vi "Get Lvm Data.vi"(8 "Error In":errorcluster, 11 "Path In":path) -> (0 "Error Out":errorcluster, 2 "Traces":T1(array[cluster]), 3 "Path Out":path)   [LabVIEW 2014, in "Aquisicao de Dados.lvlib"]
uses:
  Aquisicao de Dados.lvlib
  <vilib>/regexp/Match Regular Expression.xnode
panel:
  out "Waveform Graph":waveform(dbl)[](graph)
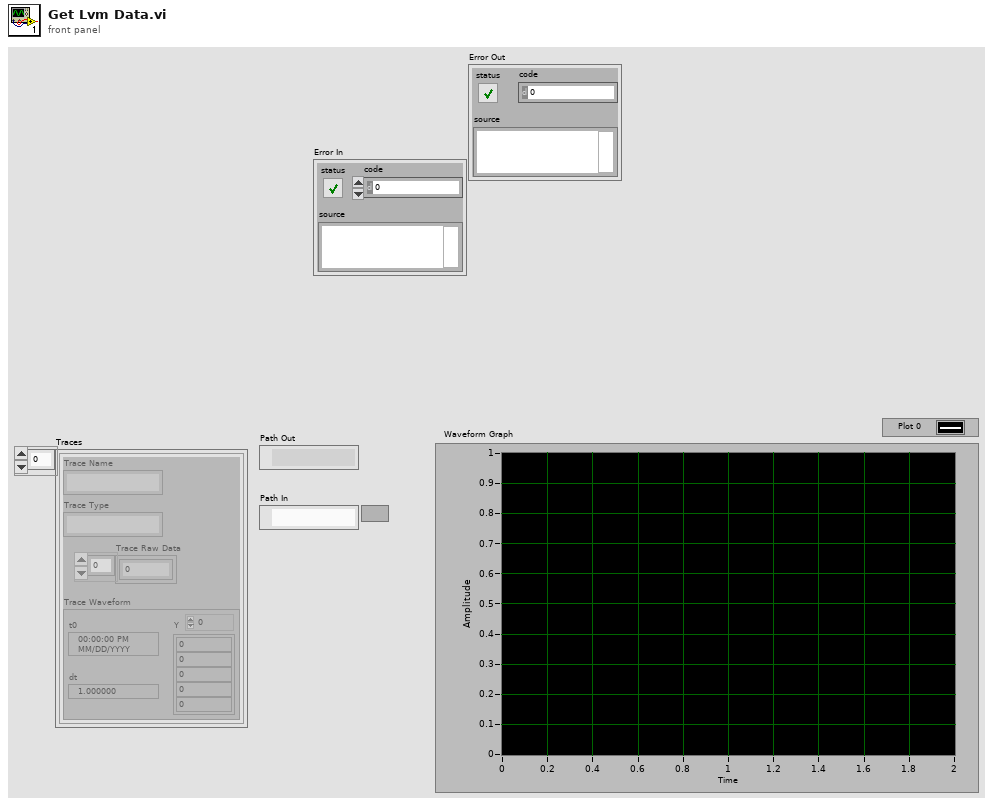
[diagram p1: front panel]
types:
  T1 = cluster{"Trace Name":string, "Trace Type":string, "Trace Raw Data":dbl[], "Trace Waveform":waveform(dbl)}[]
  T2 = cluster{"Trace Name":string, "Trace Type":string, "Trace Raw Data":dbl[], "Trace Waveform":waveform(dbl)}
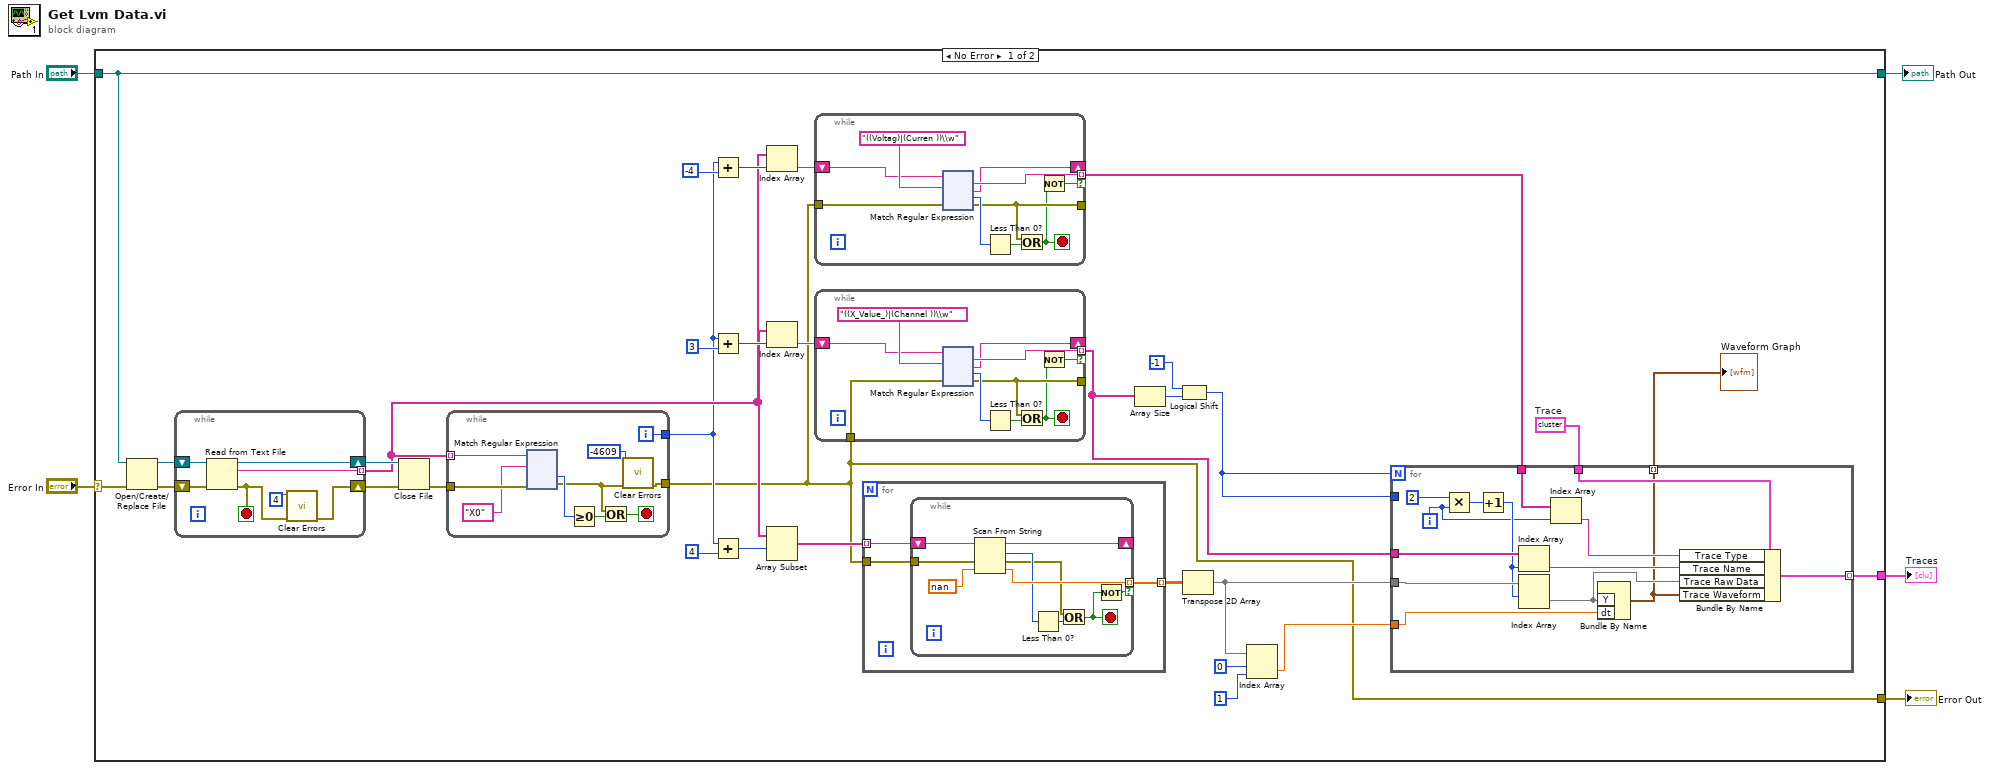
[diagram p0: block diagram]
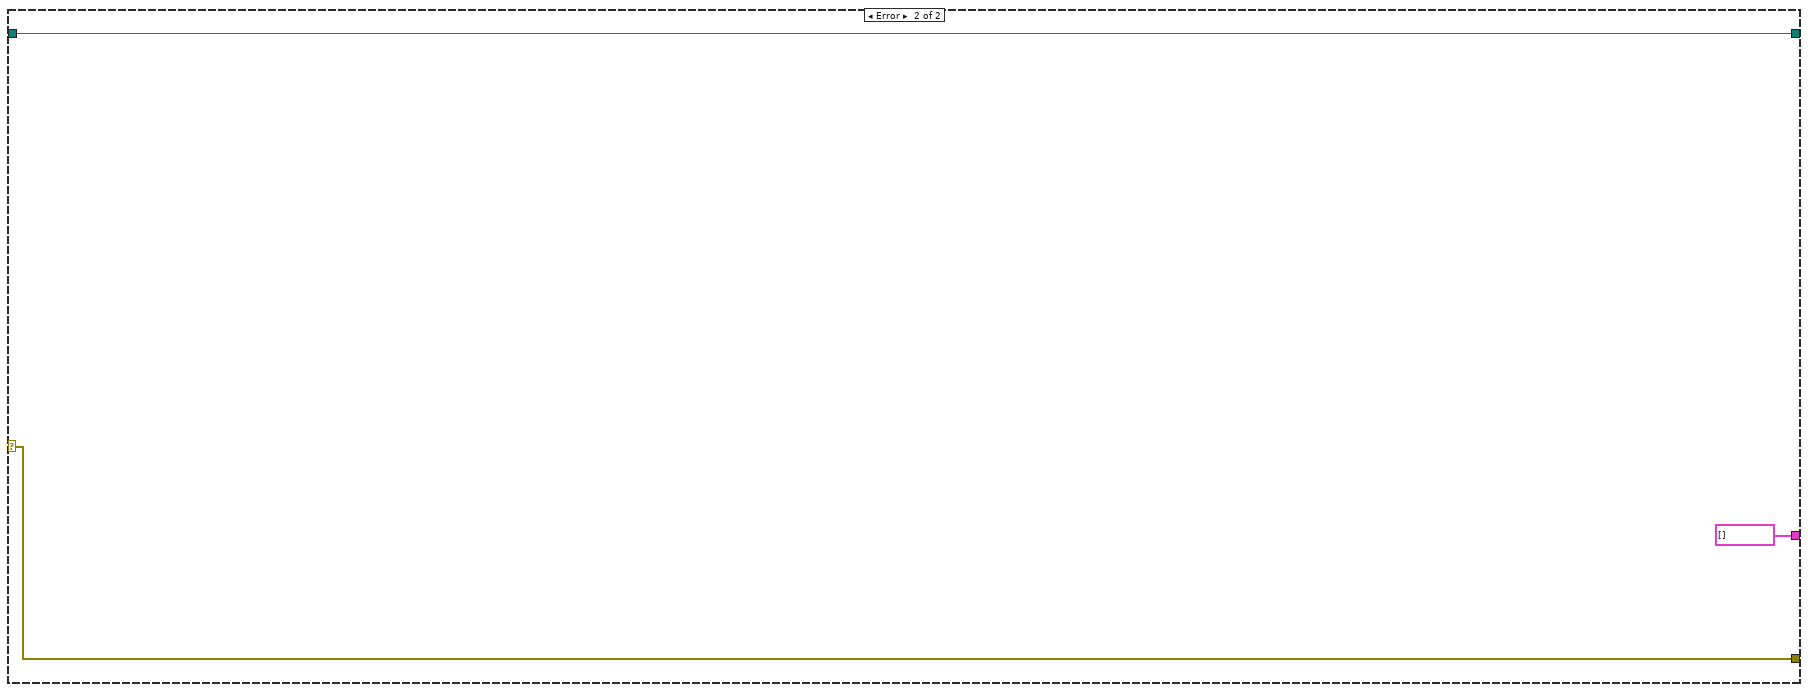
[diagram p2: hidden frame]
diagram:
  n1 = case shown="No Error" "Error In" {
    selector: "Error In" -> [w37 w444]
    tunnel: "Path In" -> [w36 w446]
    tunnel: [w36 w446] -> w3
    tunnel: [w8 T1 []] -> w2
    tunnel: [w7 w444] -> w1
    frame No Error {
      w19 = T2 {"Trace Name"="", "Trace Type"="", "Trace Raw Data"=[], "Trace Waveform"={"t0"=timestamp(0 s since 1904-01-01), "dt"=1.0, "Y"=[]}}  # Trace
      n2 = Open/Create/Replace File(file path (use dialog)=w36, error in=w37) -> (refnum out=w34:refnum<file>, error out=w35:errorcluster)  [unwired: 4 in, 1 out]
      n3 = while {
        tunnel: [w316] -> w12 mode=indexing
        shift-right: [w314] -> w33
        shift-left: w35 -> [w319]
        shift-right: [w317] -> w32
        shift-left: w34 -> [w318]
        stop <- w315 stop-if-true
        n4 = Read from Text File(file (use dialog)=w318, error in=w319) -> (refnum out=w317:refnum<file>, text=w316:string, error out=w315:errorcluster)  [unwired: 2 in, 1 out]
        n5 = call <vilib>:"Clear Errors.vi"("error in (no error)"=w315, "specific error code to clear (0: all)"=4) -> ("error out"=w314:errorcluster)  [unwired: 4 in, 1 out]
      }
      n6 = Close File(refnum=w32, error in=w33) -> (error out=w31:errorcluster)  [unwired: 1 out]
      n7 = while {
        tunnel: w12 -> [w329] mode=indexing
        tunnel: w31 -> [w328]
        tunnel: [w321] -> w7
        tunnel: [w323] -> w11
        i -> [w323]
        stop <- w326 stop-if-true
        n8 = xnode "Match Regular Expression"("input string"=w329, "regular expression"="X0", "error in"=w328) -> ("offset past match"=w324:i32, "error out"=w322:errorcluster)  [unwired: 3 in, 3 out]
        n9 = Greater Or Equal To 0?(x=w324) -> (x >= 0?=w325:bool)
        n10 = Or(x=w322, y=w325) -> (x .or. y?=w326:bool)
        n11 = call <vilib>:"Clear Errors.vi"("error in (no error)"=w322, "specific error code to clear (0: all)"=-4609) -> ("error out"=w321:errorcluster)  [unwired: 4 in, 1 out]
      }
      n12 = Add(x=w11, y=-4) -> (x+y=w14:i32)
      n13 = Add(x=w11, y=3) -> (x+y=w29:i32)
      n14 = Add(x=w11, y=4) -> (x+y=w27:i32)
      n15 = Index Array(array=w12, index=w14) -> (element=w10:string)
      n16 = Index Array(array=w12, index=w29) -> (element=w26:string)
      n17 = Array Subset(array=w12, index=w27) -> (w23:string[])  [unwired: 1 in]
      n18 = while {
        tunnel: [w43] -> _
        tunnel: [w42] -> w9 mode=indexing if=w39
        shift-right: [w41] -> _
        shift-left: w10 -> [w46]
        tunnel: w7 -> [w38]
        stop <- w40 stop-if-true
        n19 = xnode "Match Regular Expression"("input string"=w46, "regular expression"="((Voltag)|(Curren ))\\w", "error in"=w38) -> ("whole match"=w42:string, "after match"=w41:string, "offset past match"=w44:i32, "error out"=w43:errorcluster)  [unwired: 3 in, 1 out]
        n20 = Less Than 0?(x=w44) -> (x < 0?=w45:bool)
        n21 = Or(x=w43, y=w45) -> (x .or. y?=w40:bool)
        n22 = Not(x=w40) -> (.not. x?=w39:bool)
      }
      n23 = while {
        tunnel: w7 -> [w196]
        tunnel: [w193] -> _
        tunnel: [w192] -> w20 mode=indexing if=w189
        shift-right: [w191] -> _
        shift-left: w26 -> [w197]
        stop <- w190 stop-if-true
        n24 = xnode "Match Regular Expression"("input string"=w197, "regular expression"="((X_Value_)|(Channel ))\\w", "error in"=w196) -> ("whole match"=w192:string, "after match"=w191:string, "offset past match"=w194:i32, "error out"=w193:errorcluster)  [unwired: 3 in, 1 out]
        n25 = Less Than 0?(x=w194) -> (x < 0?=w195:bool)
        n26 = Or(x=w193, y=w195) -> (x .or. y?=w190:bool)
        n27 = Not(x=w190) -> (.not. x?=w189:bool)
      }
      n28 = for {
        tunnel: w23 -> [w178] mode=indexing
        tunnel: w7 -> [w177]
        tunnel: [w176] -> w22 mode=indexing
        n29 = while {
          shift-right: [w187] -> _
          shift-left: w178 -> [w188]
          tunnel: w177 -> [w186]
          tunnel: [w185] -> w176 mode=indexing if=w179
          stop <- w180 stop-if-true
          n30 = Scan From String(input string=w188, error in=w186, default 1=nan ("default value 1")) -> (remaining string=w187:string, offset past scan=w183:u32, error out=w181:errorcluster, output 1=w185:dbl)  [unwired: 2 in]
          n31 = Less Than 0?(x=w183) -> (x < 0?=w182:bool)
          n32 = Or(x=w181, y=w182) -> (x .or. y?=w180:bool)
          n33 = Not(x=w180) -> (.not. x?=w179:bool)
        }
      }
      n34 = Array Size(array=w20) -> (size(s)=w25:i32)
      n35 = Logical Shift(y=i16 -1, x=w25) -> (x << y=w21:i32)
      n36 = Transpose 2D Array(2D array=w22) -> (transposed array=w18:dbl[][])
      n37 = Index Array(array=w18, index (row)=0, index (col)=1 ("disabled index (col)")) -> (element=w15:dbl)
      n38 = for {
        N: w21 -> [_]
        tunnel: w18 -> [w172]
        tunnel: w21 -> [_]
        tunnel: w20 -> [w173]
        tunnel: w19 -> [w169]
        tunnel: w15 -> [w171]
        tunnel: w9 -> [w165]
        tunnel: [w167] -> w8 mode=indexing
        tunnel: [w162] -> w6 mode=indexing
        i -> [w163]
        n39 = Multiply(x=2, y=w163) -> (x*y=w174:i32)
        n40 = Increment(x=w174) -> (x+1=w166:i32)
        n41 = Index Array(array=w173, index=w166) -> (element=w170:string)
        n42 = Index Array(array=w172, index (row)=w166) -> (element=w168:dbl[])  [unwired: 1 in]
        n43 = Index Array(array=w165, index=w163) -> (element=w164:string)
        n44 = Bundle By Name("Y"=w168, "dt"=w171) -> (w162:waveform(dbl))  [unwired: 1 in]
        n45 = Bundle By Name(cluster=w169, "Trace Type"=w164, "Trace Name"=w170, "Trace Raw Data"=w168, "Trace Waveform"=w162) -> (w167:T2)
      }
      "Waveform Graph" <- w6
    }
    frame Error {
    }
  }
  "Path Out" <- w3
  "Traces" <- w2
  "Error Out" <- w1
